vi "Line Detection.vi"() -> ()   [LabVIEW 2018]
uses:
  <vilib>/Rock Robotics/WPI/Joystick/WPI_JoystickDevRef.ctl
  <vilib>/Rock Robotics/WPI/Joystick/WPI_JoystickDeviceEnum.ctl
  Framework/Robot Global Data.vi
  <vilib>/ptbypt/NI_PtbyPt.lvlib
panel:
  in  "JoystickDevRef":T1={"Device"=enum."USB 1"}
  in  "Robot Speed":dbl format="%#_13g"
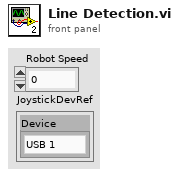
[diagram p1: front panel]
types:
  T1 = typedef "WPI_JoystickDevRef.ctl" = cluster{"Device":T2}
  T2 = typedef "WPI_JoystickDeviceEnum.ctl" = enum16{"USB 0", "USB 1", "USB 2", "USB 3", "USB 4", "USB 5"}
  T3 = typedef "WPI_SwitchDevRef.ctl" = cluster{"DevStatus":errorcluster, "DIO Channel":T4, "CntIndex":T5, "Normally Closed":bool}
  T4 = typedef "FPGA_DIOChannel.ctl" = enum8{"DIO 0", "DIO 1", "DIO 2", "DIO 3", "DIO 4", "DIO 5", "DIO 6", "DIO 7", "DIO 8", "DIO 9", "DIO MXP 0", "DIO MXP 1", "DIO MXP 2", "DIO MXP 3", "DIO MXP 4", "DIO MXP 5", "DIO MXP 6", "DIO MXP 7", "DIO MXP 8", "DIO MXP 9", "DIO MXP 10", "DIO MXP 11", "DIO MXP 12", "DIO MXP 13", "DIO MXP 14", "DIO MXP 15", "SPI Port CS1", "SPI Port CS2", "SPI Port CS3", "SPI Port MISO", "SPI Port MOSI", "Invalid"}
  T5 = typedef "FPGA_CounterCtrSystemIndex.ctl" = enum8{"Ctr 0", "Ctr 1", "Ctr 2", "Ctr 3", "Ctr 4", "Ctr 5", "Ctr 6", "Ctr 7", "Invalid"}
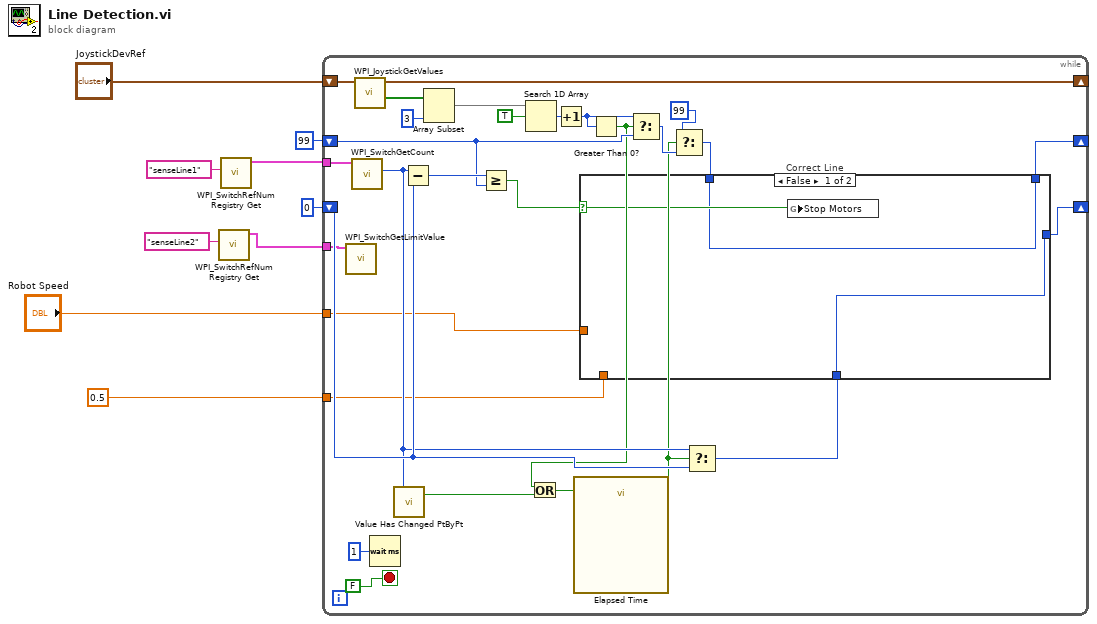
[diagram p0: block diagram]
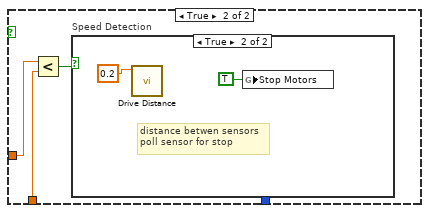
[diagram p2: hidden frame]
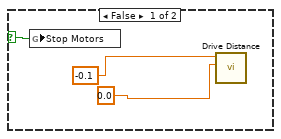
[diagram p3: hidden frame]
diagram:
  n1 = call <vilib>:"WPI_SwitchRefNum Registry Get.vi"("refnum name"="senseLine2") -> ("SwitchDevRef"=w1:T3)  [unwired: 9 in, 1 out]
  n2 = call <vilib>:"WPI_SwitchRefNum Registry Get.vi"("refnum name"="senseLine1") -> ("SwitchDevRef"=w4:T3)  [unwired: 9 in, 1 out]
  n3 = while {
    shift-right: [w35] -> _
    shift-left: "JoystickDevRef" -> [w36]
    tunnel: w4 -> [w30]
    shift-right: [w12] -> _
    shift-left: 0 ("length") -> [w28]
    shift-right: [w15] -> _
    shift-left: 99 ("length") -> [w25]
    tunnel: "Robot Speed" -> [w16]
    tunnel: 0.5 -> [w11]
    tunnel: w1 -> [w10]
    stop <- FALSE stop-if-true
    n4 = call <vilib>:"WPI_SwitchGetLimitValue.vi"("SwitchDevRef"=w10) -> ()  [unwired: 8 in, 3 out]
    n5 = call <vilib>:"WPI_SwitchGetCount.vi"("SwitchDevRef"=w30) -> ("Switch Pressed Count"=w27:i32)  [unwired: 8 in, 2 out]
    n6 = call <vilib>:"WPI_JoystickGetValues.vi"("JoystickDevRef"=w36) -> ("Buttons"=w34:bool[], "JoystickDevRef"=w35:T1)  [unwired: 6 in, 3 out]
    n7 = Wait (ms)(milliseconds to wait=u32 1) -> ()  [unwired: 1 out]
    n8 = call <vilib>:"Value Has Changed PtByPt.vi"("input data point"=w27) -> ("has changed"=w20:bool)  [unwired: 1 in, 1 out]
    n9 = Subtract(x=w27, y=w28) -> (x-y=w26:i32)
    n10 = Array Subset(array=w34, length=3) -> (w32:bool[])  [unwired: 1 in]
    n11 = Greater Or Equal?(x=w26, y=w25) -> (x >= y?=w17:bool)
    n12 = Search 1D Array(1D array=w32, element=TRUE) -> (index of element=w29:i32)  [unwired: 1 in]
    n13 = Increment(x=w29) -> (x+1=w24:i32)
    n14 = Greater Than 0?(x=w24) -> (x > 0?=w18:bool)
    n15 = Or(x=w18, y=w20) -> (x .or. y?=w19:bool)
    n16 = call "Elapsed Time"("Reset"=w19) -> ("Time has Elapsed"=w22:bool)  [unwired: 11 in, 7 out]
    n17 = Select(t=w24, s=w18, f=w25) -> (s? t:f=w23:i32)
    n18 = Select(t=99 ("length"), s=w22, f=w23) -> (s? t:f=w14:i32)
    n19 = Select(t=w27, s=w22, f=w28) -> (s? t:f=w13:i32)
    n20 = case "Correct Line" shown="False" w17 {
      selector: w17 -> [w41 _]
      tunnel: w16 -> [_ w44]
      tunnel: [w40 _] -> w15
      tunnel: w14 -> [w40 _]
      tunnel: [w39 _] -> w12
      tunnel: w13 -> [w39 _]
      tunnel: w11 -> [_ w42]
      frame False {
        n21 = global write "Robot Global Data.vi" "Stop Motors"(w41) -> ()
      }
      frame True {
        n22 = Less?(x=w44, y=w42) -> (x < y?=w43:bool)
        n23 = case "Speed Detection" shown="True" w43 {
          selector: w43 -> [w47 _]
          frame False {
            n24 = global write "Robot Global Data.vi" "Stop Motors"(w47) -> ()
            n25 = call "Drive Distance.vi"("Distance"=0.0, "Speed"=-0.1) -> ()  [unwired: 9 in, 1 out]
          }
          frame True {
            # "distance betwen sensors\npoll sensor for stop"
            n26 = call "Drive Distance.vi"("Speed"=0.2) -> ()  [unwired: 10 in, 1 out]
            n27 = global write "Robot Global Data.vi" "Stop Motors"(TRUE ("Stop Motors")) -> ()
          }
        }
      }
    }
  }
